vi "Session Event Callback.vi"(4 "Session User Event":refnum<user-event>, 5 "Event Data":cluster{"sender":refnum<k24>, "e":refnum<k24>}, 6 "Session Ref":T1, 7 "Event Common Data":T2) -> ()   [LabVIEW 2020, in "NI_VS Sequence Execution Interface.lvlib"]
uses:
  <vilib>/NI VeriStand/Execution/SequenceExecutionInterface/NI_VS Sequence Execution Interface.lvlib
  <vilib>/NI VeriStand/Execution/SequenceExecutionInterface/Stimulus Profile Session Ref.ctl
  NationalInstruments.VeriStand.ClientAPI
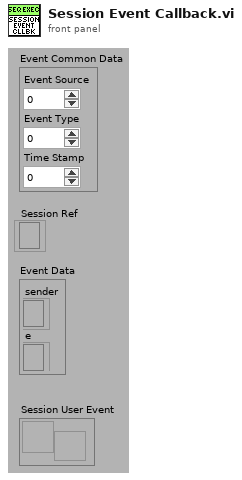
[diagram p1: front panel]
types:
  T1 = typedef "NI_VS Sequence Execution Interface.lvlib/Stimulus Profile Session Ref.ctl" = refnum<k24>
  T2 = cluster{"Event Source":i32, "Event Type":u32, "Time Stamp":u32}
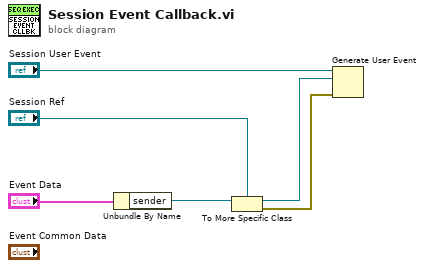
[diagram p0: block diagram]
diagram:
  n1 = Unbundle By Name("Event Data") -> ("sender"=w4:refnum<k24>)
  n2 = To More Specific Class(target class="Session Ref", reference=w4) -> (specific class reference=w1:T1, error out=w6:errorcluster)  [unwired: 1 in]
  n3 = Generate User Event(user event="Session User Event", event data cluster=w1, error in=w6) -> ()  [unwired: 1 in, 2 out]
